vi "U8 Array.vi"(8 "Error In":errorcluster) -> (0 "Error Out":errorcluster)   [LabVIEW 2018, in "Tests.lvlib" / "From Msgpack.lvlib"]
uses:
  From Msgpack.lvlib
  <vilib>/addons/_JKI Toolkits/Caraya/classes/Test/Test.lvclass
  src/Toolkit/Toolkit.lvlib
  <vilib>/addons/_JKI Toolkits/Caraya/classes/Assert/Assert.lvclass
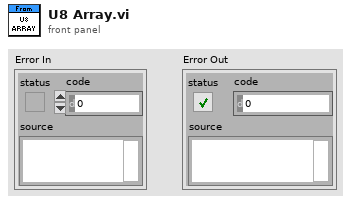
[diagram p1: front panel]
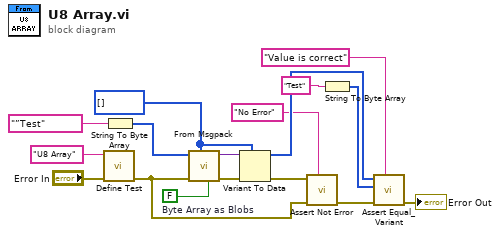
[diagram p0: block diagram]
diagram:
  w3 = u8[] []
  w4 = FALSE  # Byte Array as Blobs
  n1 = call <vilib>:"Define Test.vi"("error in (no error)"="Error In", "Label (VI Title)"="U8 Array") -> ("error out"=w11:errorcluster)  [unwired: 9 in]
  n2 = String To Byte Array(string="”Test") -> (unsigned byte array=w14:u8[])
  n3 = call "From Msgpack.vi"("Byte Array as Blobs"=w4, "Types and Defaults"=w3, "Error In"=w11, "Msgpack Data"=w14) -> ("Error Out"=w15:errorcluster, "Value"=w13:variant)  [unwired: 6 in]
  n4 = Variant To Data(error in=w15, type=w3, Variant=w13) -> (data=w8:u8[], error out=w12:errorcluster)
  n5 = call <vilib>:"Assert Not Error.vi"("Label"="No Error", "error in (no error)"=w11, "Not Error?"=w12) -> ("error out"=w10:errorcluster)  [unwired: 8 in]
  n6 = String To Byte Array(string="Test") -> (unsigned byte array=w1:u8[])
  n7 = call <vilib>:"Assert Equal_Variant.vi"("Label"="Value is correct", "error in (no error)"=w10, "Y"=w1, "X"=w8) -> ("error out"=→"Error Out":errorcluster)  [unwired: 7 in]
